vi "Manipulation1.vi"() -> ()   [LabVIEW 2017]
panel:
  out "Moyenne de classe":dbl
  out "Mauvaise Moyenne":dbl
  out "Meilleure Moyenne":dbl
  out "Moyenne":dbl[](array[numeric])
  in  "Examan":dbl[](array[numeric])
  in  "DS":dbl[](array[numeric])
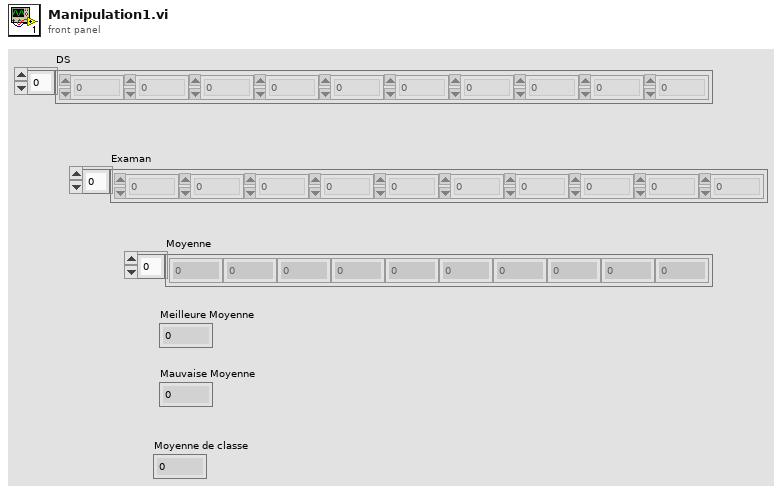
[diagram p1: front panel]
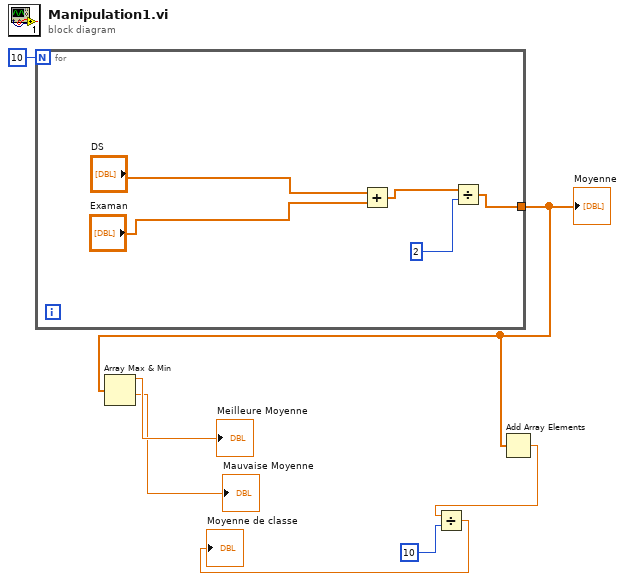
[diagram p0: block diagram]
diagram:
  n1 = for {
    N: 10 -> [_]
    tunnel: [w10] -> w4
    n2 = Add(x="DS", y="Examan") -> (x+y=w11:dbl[])
    n3 = Divide(x=w11, y=2) -> (x/y=w10:dbl[])
  }
  "Moyenne" <- w4
  n4 = Array Max & Min(array=w4) -> (max value=→"Meilleure Moyenne":dbl, min value=→"Mauvaise Moyenne":dbl)  [unwired: 2 out]
  n5 = Add Array Elements(numeric array=w4) -> (sum=w3:dbl)
  n6 = Divide(x=w3, y=10) -> (x/y=→"Moyenne de classe":dbl)
